vi "mupExpr Calc.vi"() -> ()   [LabVIEW 2015]
uses:
  mupExpr/mupExpr.lvclass/mupExpr.ctl
  mupExpr/Eval_SglRes.vi
  mupLib/mupEval.vi
  mupLib/mupCheckError.vi
  mupLib/mupLibPath.vi
  <vilib>/Utility/error.llb/Error Cluster From Error Code.vi
  mupExpr/mupExpr.lvclass
panel:
  out "Result":dbl=nan format="%#_20g"
  out "error out":errorcluster
  in  "Expression":string="0"
  in  "Calculate":bool
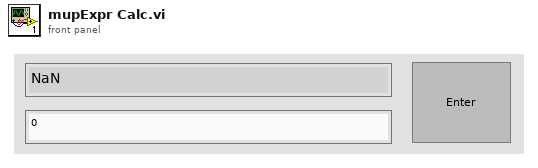
[diagram p1: front panel]
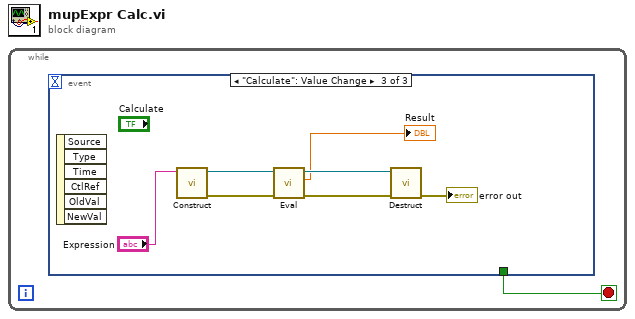
[diagram p0: block diagram]
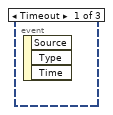
[diagram p2: hidden frame]
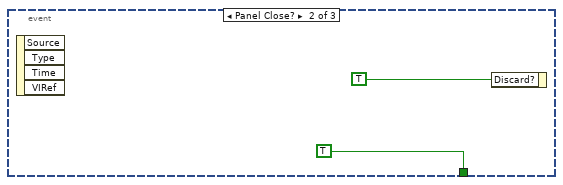
[diagram p3: hidden frame]
diagram:
  n1 = while {
    stop <- w1 stop-if-true
    n2 = event shown="[2] \"Calculate\": Value Change" {
      selector: _ -> [_ _ _]
      dyn-events: _ -> [_ _ _]
      timeout: _ -> [_ _ _]
      tunnel: [_ TRUE _] -> w1
      event Timeout {
        n3 = event-data() -> ()  [unwired: 1 in, 3 out]
      }
      event Panel Close? {
        n4 = event-data() -> ()  [unwired: 1 in, 4 out]
        n5 = event-data("Discard?"=TRUE) -> ()  [unwired: 1 in, 1 out]
      }
      event "Calculate": Value Change {
        n6 = event-data() -> ()  [unwired: 1 in, 6 out]
        n7 = call "Construct.vi"("Expression"="Expression") -> ("error out"=w9:errorcluster, "mupExpr out"=w7:refnum<data-value>)  [unwired: 8 in, 1 out]
        n8 = call-poly "Eval.vi"("error in (no error)"=w9, "mupExpr in"=w7) -> ("error out"=w10:errorcluster, "Result"=→"Result":dbl, "mupExpr out"=w8:refnum<data-value>)  [unwired: 7 in]
        n9 = call "Destruct.vi"("error in (no error)"=w10, "mupExpr in"=w8) -> ("error out"=→"error out":errorcluster)  [unwired: 9 in]
      }
    }
  }
